vi "Find Result File Directory.vi"(8 "error in (no error)":errorcluster, 10 "Directory Name":string="Results", 11 "Parent Path":path) -> (0 "error out":errorcluster, 3 "Result Directory":path)   [LabVIEW 2016]
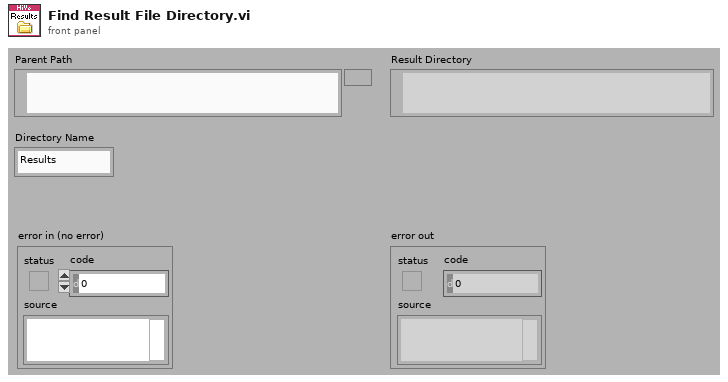
[diagram p1: front panel]
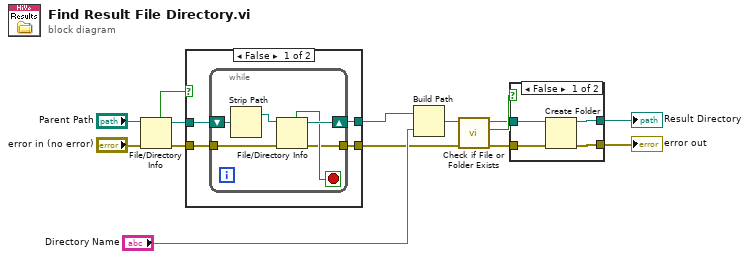
[diagram p0: block diagram]
diagram:
  n1 = File/Directory Info(path="Parent Path", error in="error in (no error)") -> (path out=w2:path, directory=w1:bool, error out=w4:errorcluster)  [unwired: 4 out]
  n2 = case shown="False" w1 {
    tunnel: [w18 w26] -> w14
    tunnel: w4 -> [w17 w25]
    tunnel: [w16 w25] -> w11
    tunnel: w2 -> [w15 w26]
    frame False {
      n3 = while {
        shift-right: [w23] -> w18
        shift-left: w15 -> [w21]
        tunnel: [w20] -> w16
        tunnel: w17 -> [w19]
        stop <- w22 stop-if-true
        n4 = Strip Path(path=w21) -> (stripped path=w24:path)  [unwired: 1 out]
        n5 = File/Directory Info(path=w24, error in=w19) -> (path out=w23:path, directory=w22:bool, error out=w20:errorcluster)  [unwired: 4 out]
      }
    }
    frame True {
    }
  }
  n6 = Build Path(base path=w14, name or relative path="Directory Name") -> (appended path=w10:path)
  n7 = call <vilib>:"Check if File or Folder Exists.vi"("error in (no error)"=w11, "path"=w10) -> ("error out"=w9:errorcluster, "file or folder exists?"=w8:bool, "dup path"=w7:path)  [unwired: 7 in]
  n8 = case shown="False" w8 {
    tunnel: w7 -> [w30 w32]
    tunnel: [w29 w32] -> w6
    tunnel: w9 -> [w28 w31]
    tunnel: [w27 w31] -> w12
    frame False {
      n9 = Create Folder(path (use dialog)=w30, error in=w28) -> (created path=w29:path, error out=w27:errorcluster)  [unwired: 1 in, 1 out]
    }
    frame True {
    }
  }
  "error out" <- w12
  "Result Directory" <- w6
